vi "Reorder Points.vi"(10 "Y":dbl[](array[numeric]), 11 "X":dbl[](array[numeric])) -> (2 "Y'":dbl[](array[numeric]), 3 "X'":dbl[](array[numeric]))   [LabVIEW 2021, in "d15.lvlib" / "Diamond.lvclass"]
uses:
  Diamond.lvclass
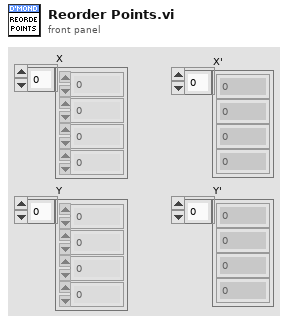
[diagram p1: front panel]
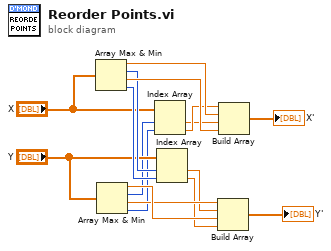
[diagram p0: block diagram]
diagram:
  n1 = Array Max & Min(array="X") -> (max value=w13:dbl, max index (indices)=w7:i32, min value=w14:dbl, min index (indices)=w8:i32)
  n2 = Array Max & Min(array="Y") -> (max value=w16:dbl, max index (indices)=w3:i32, min value=w15:dbl, min index (indices)=w5:i32)
  n3 = Index Array(array="X", index #1=w3, index #2=w5) -> (element #1=w1:dbl, element #2=w4:dbl)
  n4 = Index Array(array="Y", index #1=w7, index #2=w8) -> (element #1=w9:dbl, element #2=w10:dbl)
  n5 = Build Array(w15, w9, w16, w10) -> (→"Y'":dbl[])
  n6 = Build Array(w4, w13, w1, w14) -> (→"X'":dbl[])
